vi "Fetch Waveform (Waveform Data Type)_mod.vi"(4 "Save data":bool, 6 "Channel name to save":string, 7 "tdms file":refnum<k34>, 8 "error in (no error)":errorcluster, 9 "Maximum Time (10000ms)":u32=10000, 10 "Channel (0: Channel 1)":u16(ring) items=["Channel 1", "Channel 2", "Channel 3", "Channel 4", "Math", "Reference 1", "Reference 2", "Reference 3", "Reference 4", "D0", "D1", "D2", "D3", "D4", "D5", "D6", "D7", "D8", "D9", "D10", "D11", "D12", "D13", "D14", "D15", "Amplitude", "Frequency", "Phase", "Normal", "Average", "Maximum Peak Hold", "Minimum Peak Hold"], 11 "VISA resource name":refnum<visa-resource-name>) -> (0 "error out":errorcluster, 2 "Waveform Data":waveform(dbl)(graph), 3 "VISA resource name out":refnum<visa-resource-name>, 5 "tdms file out":refnum<k34>)   [LabVIEW 2015]
doc: "Returns the waveform that an oscilloscope acquires for a channel you specify. An acquisition that you initiate before calling this VI generates the waveform.\n\nYou first enable channels with the Configure Channel VI. Then you use the Initiate VI to start an acquisition on the enabled channels. An oscilloscope concurrently acquires waveforms for these channels. You must call the Fetch Waveform VI separately to obtain waveforms for each enabled channel.\nHowever, you also can call the Read Waveform VI instead of using the above low-level VIs.\n\n<B>Note</B>: Use the Fetch Waveform VI only with other low-level VIs, such as the Initiate VI, the Abort VI, and the Fetch Waveform Measurement VI. High-level VIs, such as the Read Waveform VI, automatically incorporate the functions of the Initiate VI and the Fetch Waveform VI. The Fetch Waveform VI does not check the status of an instrument."
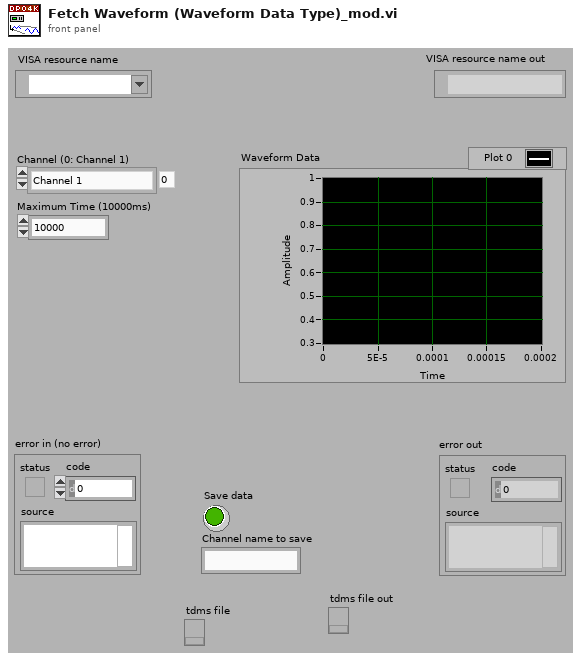
[diagram p1: front panel]
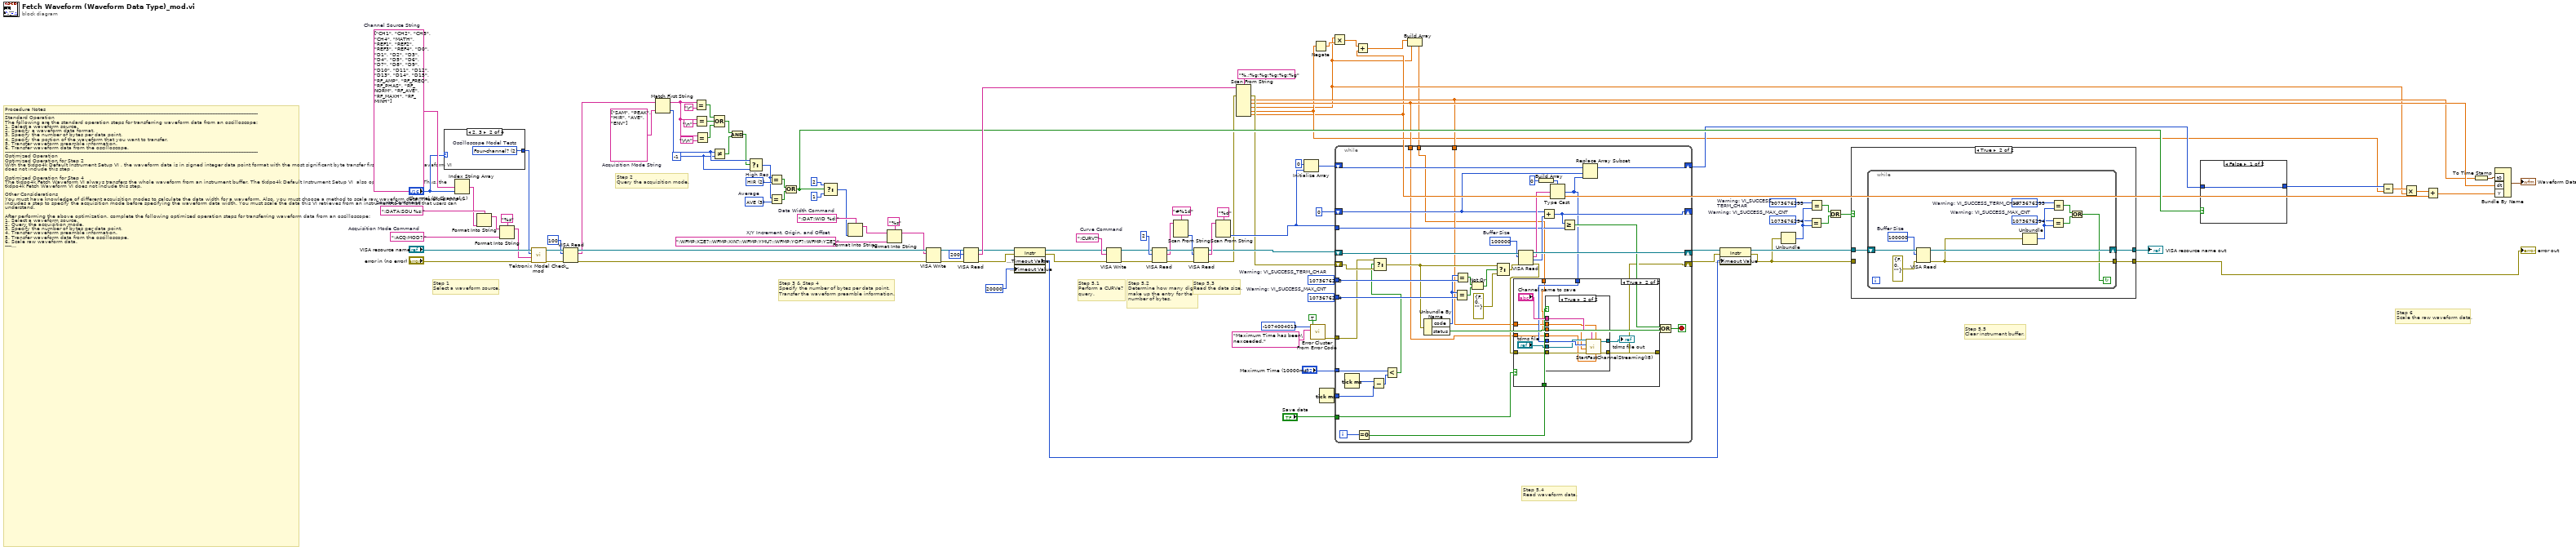
[diagram p0: block diagram]
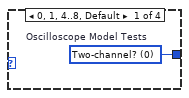
[diagram p2: hidden frame]
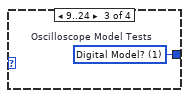
[diagram p3: hidden frame]
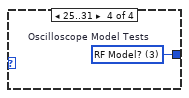
[diagram p4: hidden frame]
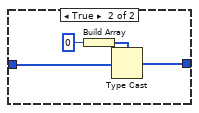
[diagram p5: hidden frame]
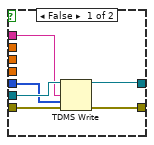
[diagram p8: hidden frame]
diagram:
  w51 = 1073676294  # Warning: VI_SUCCESS_MAX_CNT
  w52 = 1073676293  # Warning: VI_SUCCESS_TERM_CHAR
  w55 = 1073676294  # Warning: VI_SUCCESS_MAX_CNT
  w54 = 1073676293  # Warning: VI_SUCCESS_TERM_CHAR
  w64 = -1 ("y")
  w89 = ":CURV?"  # Curve Command
  w99 = ":DAT:WID %d;"  # Data Width Command
  w104 = u16 3 items=["SAM", "PEAK", "HIR", "AVE", "ENV"]  # Average
  w105 = u16 2 items=["SAM", "PEAK", "HIR", "AVE", "ENV"]  # High Res
  w76 = string[] ["SAM", "PEAK", "HIR", "AVE", "ENV"]  # Acquisition Mode String
  w98 = ":ACQ:MOD?;"  # Acquisition Mode Command
  w110 = string[] ["CH1", "CH2", "CH3", "CH4", "MATH", "REF1", "REF2", "REF3", "REF4", "D0", "D1", "D2", "D3", "D4", "D5", "D6", "D7", "D8", "D9", "D10", "D11", "D12", "D13", "D14", "D15", "RF_AMP", "RF_FREQ", "RF_PHAS", "RF_NORM", "RF_AVE", "RF_MAXH", "RF_MINH"]  # Channel Source String
  w109 = ":DATA:SOU %s;"  # Source Command
  w96 = ":WFMP:XZE?;:WFMP:XIN?;:WFMP:YMU?;:WFMP:YOF?;:WFMP:YZE?;"  # X/Y Increment, Origin, and Offset
  # "Step 6    \nScale the raw waveform data."
  # "Step 5.5    \nClear instrument buffer."
  # "Step 5.4   \nRead waveform data."
  # "Step 5.3      \nRead the data size."
  # "Step 5.2      \nDetermine how many digits\nmake up the entry for the \nnumber of bytes."
  # "Step 5.1      \nPerform a CURVe?\nquery."
  # "Step 3 & Step 4         \nSpecify the number of bytes per data point.\nTransfer the waveform preamble information."
  # "Step 2        \nQuery the acquisition mode."
  # "Step 1 \nSelect a waveform source."
  # "Procedure Notes\n-----------------------------------------------------------------------------------------------------------------------------------------------------------\nStandard Operation\nThe following are the standard operation steps for transferring waveform data from an oscilloscope:\n1. Select a waveform source.\n2. Specify a waveform data format.\n3. Specify the number of bytes per data point.\n4. Specify the portion of the waveform that you want to transfer.\n5. Transfer waveform preamble information.\n6. Transfer waveform data from the oscilloscope.\n-----------------------------------------------------------------------------------------------------------------------------------------------------------\nOptimized Operation\nOptimized Operation for Step 2\nWith the tkdpo4k Default Instrument Setup VI , the waveform data is in signed integer data point format with the most significant byte transfer first. Thus, the Fetch Waveform VI does not include this step . \n\nOptimized Operation for Step 4 \nThe tkdpo4k Fetch Waveform VI always transfers the whole waveform from an instrument buffer. The tkdpo4k Default Instrument Setup VI  also operates in this way. Thus, the tkdpo4k Fetch Waveform VI does not include this step. \n\nOther Considerations\nYou must have knowledge of different acquisition modes to calculate the data width for a waveform. Also, you must choose a method to scale raw waveform data. Therefore, this VI includes a step to specify the acquisition mode before specifying the waveform data width. You must scale the data this VI retrieves from an instrument to a format that users can understand.\n\nAfter performing the above optimization, complete the following optimized operation steps for transferring waveform data from an oscilloscope:\n1. Select a waveform source.\n2. Query the acquisition mode.\n3. Specify the number of bytes per data point.\n4. Transfer waveform preamble information.\n5. Transfer waveform data from the oscilloscope.\n6. Scale raw waveform data.\n-----------------------------------------------------------------------------------------------------------------------------------------------------------\nDetailed Steps\nThe following steps detail the behavior of this VI:\n1. Select a waveform source. \n2. Query and determine the acquisition mode. A correct determination is critical to steps 3 and 6.\n    -----------------------------------------------\n    Acquisition Mode |  Data Width   \n    -----------------------------------------------\n    Normal                       |   1                      \n    -----------------------------------------------\n    Peak Detect               |   1                      \n    -----------------------------------------------\n    Hi Res                        |   2                      \n    -----------------------------------------------\n    Envelope                   |   1                      \n    ----------------------------------------------- \n    Average                    |   2                      \n    -----------------------------------------------\n3. Specify the number of bytes per data point. For the Hi Res or Average acquisition modes, set the data width to 2. For all other acquisition modes, set the data width to 1.\n4. Transfer the waveform preamble information. Necessary preamble information includes XZero, XIncrement, YMultiplier, YOffset, and YZero. This VI uses XZero and XIncrement to configure the x-axis of output waveforms and uses YMultiplier, YOffset, and YZero to scale data values. This VI then parses the return string of the preamble query in step 6.\n5. Transfer waveform data from the oscilloscope.\n    5.1 Perform a CURVe? query.\n    5.2 Determine how many digits make up the entry for the number of bytes.\n    5.3 Read the data size.\n    5.4 Call the VISA Read VI repeatedly with a buffer size of 10000 until you obtain as much data as the data size specifies. Use      an 8-bit array to store the raw waveform data you obtain. \n    5.5 Continue reading the data remaining in the instrument buffer until the buffer is empty.\n6. Scale the raw waveform data.\n    6.1 Cast the waveform data to a 16-bit array if the data width is 2 . Split the waveform data into a minimum and a maximum data array if the acquisition mode is Peak Detect or Envelope. This VI skips this step if the data width is 1.\n    6.2 Parse the preamble information.\n    6.3 Scale the waveform data according to the following formula:\n          Data_Value_in_units = (Raw_Data_Value - YOffset) * YMultiplier + YZero\n          The resulting waveform data has a unit of volts.\n    6.4 Build a waveform graph."
  n1 = case shown="2, 3" "Channel (0: Channel 1)" {
    tunnel: [w111 w112 w113 w114] -> w14
    frame 0, 1, 4..8, Default {
      w111 = u16 0 items=["Two-channel?", "Digital Model?", "Four-channel?", "RF Model?"]  # Oscilloscope Model Tests
    }
    frame 2, 3 {
      w112 = u16 2 items=["Two-channel?", "Digital Model?", "Four-channel?", "RF Model?"]  # Oscilloscope Model Tests
    }
    frame 9..24 {
      w113 = u16 1 items=["Two-channel?", "Digital Model?", "Four-channel?", "RF Model?"]  # Oscilloscope Model Tests
    }
    frame 25..31 {
      w114 = u16 3 items=["Two-channel?", "Digital Model?", "Four-channel?", "RF Model?"]  # Oscilloscope Model Tests
    }
  }
  n2 = Index String Array(1:"Channel (0: Channel 1)", 2:w110) -> (0:w108:string)  [unwired: 1 in]
  n3 = Format Into String(format string=w109, w108) -> (resulting string=w107:string)  [unwired: 2 in, 1 out]
  n4 = Format Into String(format string="%s", initial string=w107, w98) -> (resulting string=w19:string)  [unwired: 1 in, 1 out]
  n5 = call "Tektronix Model Check_mod.vi"("error in (no error)"="error in (no error)", "Command String"=w19, "Oscilloscope Model Tests (3: RF Model?)"=w14, "VISA resource name"="VISA resource name") -> ("error out"=w17:errorcluster, "VISA resource name out"=w18:refnum<visa-resource-name>)  [unwired: 6 in]
  n6 = VISA Read(VISA resource name=w18, byte count=u32 100, error in (no error)=w17) -> (VISA resource name out=w95:refnum<visa-resource-name>, read buffer=w75:string, error out=w94:errorcluster)  [unwired: 1 out]
  n7 = Match First String(2:w76, 3:w75) -> (0:w65:i32, 1:w71:string)
  n8 = Equal?(x=w71, y="\r") -> (x = y?=w70:bool)
  n9 = Equal?(x=w71, y="\n") -> (x = y?=w69:bool)
  n10 = Equal?(x=w71, y="\r\n") -> (x = y?=w68:bool)
  n11 = Not Equal?(x=w65, y=w64) -> (x != y?=w66:bool)
  n12 = Compound Arithmetic op=OR(w70, w69, w68) -> (w67:bool)
  n13 = And(x=w67, y=w66) -> (x .and. y?=w63:bool)
  n14 = Select(t=w65, s=w63, f=w64) -> (s? t:f=w50:i32)
  n15 = Equal?(x=w50, y=w105) -> (x = y?=w103:bool)
  n16 = Equal?(x=w50, y=w104) -> (x = y?=w102:bool)
  n17 = Or(x=w103, y=w102) -> (x .or. y?=w49:bool)
  n18 = Select(t=2 ("f"), s=w49, f=1) -> (s? t:f=w79:i32)
  n19 = Format Into String(format string=w99, w79) -> (resulting string=w93:string)  [unwired: 2 in, 1 out]
  n20 = Format Into String(format string="%s", initial string=w93, w96) -> (resulting string=w80:string)  [unwired: 1 in, 1 out]
  n21 = VISA Write(VISA resource name=w95, write buffer=w80, error in (no error)=w94) -> (VISA resource name out=w91:refnum<visa-resource-name>, error out=w90:errorcluster)  [unwired: 1 out]
  n22 = VISA Read(VISA resource name=w91, byte count=u32 200, error in (no error)=w90) -> (VISA resource name out=w28:refnum<visa-resource-name>, read buffer=w78:string, error out=w27:errorcluster)  [unwired: 1 out]
  n23 = property class="Instr"(reference=w28, error in=w27, "General Settings:Timeout Value"=u32 20000) -> (reference out=w26:refnum<visa-resource-name>, error out=w24:errorcluster, "General Settings:Timeout Value"=w37:u32)
  n24 = VISA Write(VISA resource name=w26, write buffer=w89, error in (no error)=w24) -> (VISA resource name out=w25:refnum<visa-resource-name>, error out=w23:errorcluster)  [unwired: 1 out]
  n25 = VISA Read(VISA resource name=w25, byte count=u32 2, error in (no error)=w23) -> (VISA resource name out=w86:refnum<visa-resource-name>, read buffer=w84:string, error out=w85:errorcluster)  [unwired: 1 out]
  n26 = Scan From String(format string="#%1d", input string=w84) -> (output 1=w83:i32)  [unwired: 3 in, 3 out]
  n27 = VISA Read(VISA resource name=w86, byte count=w83, error in (no error)=w85) -> (VISA resource name out=w22:refnum<visa-resource-name>, read buffer=w81:string, error out=w11:errorcluster)  [unwired: 1 out]
  n28 = Scan From String(format string="%d", input string=w81) -> (output 1=w62:i32)  [unwired: 3 in, 3 out]
  n29 = Scan From String(format string="%.;%g;%g;%g;%g;%g", input string=w78, error in=w11) -> (error out=w10:errorcluster, output 1=w8:dbl, output 2=w9:dbl, output 3=w2:dbl, output 4=w6:dbl, output 5=w4:dbl)  [unwired: 6 in, 2 out]
  n30 = Initialize Array(i8 0 ("element"), w62) -> (w60:i8[])
  n31 = call <vilib>:"Error Cluster From Error Code.vi"("show call chain? (False)"=TRUE, "error message (\"\")"="Maximum Time has been\nexceeded." ("error message (\"\")"), "error code (0)"=-1074004013) -> ("error out"=w29:errorcluster)  [unwired: 6 in]
  n32 = Negate(x=w6) -> (-x=w7:dbl)
  n33 = Tick Count (ms)() -> (millisecond timer value=w34:u32)
  n34 = Multiply(x=w2, y=w7) -> (x*y=w5:dbl)
  n35 = Add(x=w5, y=w4) -> (x+y=w3:dbl)
  n36 = Build Array(w3, w2) -> (w1:dbl[])
  n37 = while {
    shift-right: [w152] -> w39
    shift-left: w22 -> [w154]
    shift-right: [w119] -> w38
    shift-left: w10 -> [w126]
    shift-right: [w148] -> w48
    shift-left: w60 -> [w149]
    tunnel: w62 -> [w145]
    shift-right: [w143] -> _
    shift-left: 0 -> [w144]
    tunnel: w52 -> [w137]
    tunnel: w51 -> [w136]
    tunnel: w34 -> [w130]
    tunnel: "Maximum Time (10000ms)" -> [w128]
    tunnel: w29 -> [w125]
    tunnel: "Save data" -> [w121]
    tunnel: w9 -> [w117]
    tunnel: w8 -> [w116]
    tunnel: w1 -> [w115]
    i -> [w123]
    stop <- w142 stop-if-true
    w153 = 100000  # Buffer Size
    n38 = Tick Count (ms)() -> (millisecond timer value=w131:u32)
    n39 = Equal To 0?(x=w123) -> (x = 0?=w122:bool)
    n40 = Subtract(x=w131, y=w130) -> (x-y=w129:u32)
    n41 = Less?(x=w128, y=w129) -> (x < y?=w124:bool)
    n42 = Select(t=w125, s=w124, f=w126) -> (s? t:f=w127:errorcluster)
    n43 = Unbundle By Name(w127) -> ("code"=w135:i32, "status"=w139:bool)
    n44 = Equal?(x=w135, y=w136) -> (x = y?=w133:bool)
    n45 = Equal?(x=w135, y=w137) -> (x = y?=w134:bool)
    n46 = Not Or(1:w133, 2:w134) -> (0:w132:bool)
    n47 = Select(t=w127, s=w132, f=errorcluster {"status"=FALSE, "code"=0, "source"=""} ("error in (no error)")) -> (s? t:f=w138:errorcluster)
    n48 = VISA Read(VISA resource name=w154, byte count=w153, error in (no error)=w138) -> (VISA resource name out=w152:refnum<visa-resource-name>, read buffer=w147:string, return count=w146:u32, error out=w120:errorcluster)
    n49 = Build Array(i8 0) -> (w151:i8[])
    n50 = Add(x=w144, y=w146) -> (x+y=w143:u32)
    n51 = Type Cast(type=w151, x=w147) -> (*(type *) &x=w118:i8[])
    n52 = case shown="True" w121 {
      tunnel: w122 -> [_ w164]
      tunnel: w120 -> [w155 w163]
      tunnel: [w155 w162] -> w119
      tunnel: w118 -> [_ w160]
      tunnel: w117 -> [_ w159]
      tunnel: w116 -> [_ w158]
      tunnel: w115 -> [_ w157]
      frame False {
      }
      frame True {
        n53 = case shown="True" w164 {
          tunnel: w163 -> [w171 w180]
          tunnel: [w170 w179] -> w162
          tunnel: w160 -> [w166 w178]
          tunnel: "tdms file" -> [w169 w177]
          tunnel: "Channel name to save" -> [w167 w176]
          tunnel: w158 -> [_ w175]
          tunnel: w159 -> [_ w174]
          tunnel: w157 -> [_ w173]
          tunnel: [w168 w172] -> w156
          frame False {
            n54 = TDMS Write(0:w169, 7:w167, 9:w166, 11:w171) -> (4:w168:refnum<k34>, 15:w170:errorcluster)  [unwired: 2 in, 2 out]
          }
          frame True {
            n55 = call "StartFastChannelStreaming(I8).vi"("dt"=w174, "t0"=w175, "channel name(s) in (Untitled)"=w176, "error in (no error)"=w180, "Scaling coefficients"=w173, "Data"=w178, "tdms file"=w177) -> ("error out"=w179:errorcluster, "tdms file out"=w172:refnum<k34>)  [unwired: 3 in]
          }
        }
        "tdms file out" <- w156
      }
    }
    n56 = Greater Or Equal?(x=w143, y=w145) -> (x >= y?=w141:bool)
    n57 = Replace Array Subset(array=w149, new element=w118, index=w144) -> (w148:i8[])
    n58 = Compound Arithmetic op=OR(w141, w139) -> (w142:bool)
  }
  n59 = property class="Instr"(reference=w39, error in=w38, "General Settings:Timeout Value"=w37) -> (reference out=w36:refnum<visa-resource-name>, error out=w35:errorcluster)
  n60 = Unbundle(w35) -> ("code"=w56:i32)  [unwired: 2 out]
  n61 = Equal?(x=w55, y=w56) -> (x = y?=w58:bool)
  n62 = Equal?(x=w54, y=w56) -> (x = y?=w59:bool)
  n63 = Or(x=w59, y=w58) -> (x .or. y?=w57:bool)
  n64 = case shown="True" w57 {
    tunnel: w36 -> [w182 w185]
    tunnel: w35 -> [w181 _]
    tunnel: [w182 w184] -> w77
    tunnel: [w181 w183] -> w12
    frame False {
    }
    frame True {
      n65 = while {
        shift-right: [w195] -> w184
        shift-left: w185 -> [w196]
        tunnel: [w188] -> w183
        stop <- w187 continue-if-true
        w190 = 1073676294  # Warning: VI_SUCCESS_MAX_CNT
        w189 = 1073676293  # Warning: VI_SUCCESS_TERM_CHAR
        w194 = u32 100000  # Buffer Size
        n66 = VISA Read(VISA resource name=w196, byte count=w194, error in (no error)=errorcluster {"status"=FALSE, "code"=0, "source"=""}) -> (VISA resource name out=w195:refnum<visa-resource-name>, error out=w188:errorcluster)  [unwired: 2 out]
        n67 = Unbundle(w188) -> ("code"=w191:i32)  [unwired: 2 out]
        n68 = Equal?(x=w190, y=w191) -> (x = y?=w192:bool)
        n69 = Equal?(x=w189, y=w191) -> (x = y?=w193:bool)
        n70 = Or(x=w193, y=w192) -> (x .or. y?=w187:bool)
      }
    }
  }
  "error out" <- w12
  "VISA resource name out" <- w77
  n71 = case shown="False" w49 {
    tunnel: w48 -> [w197 w199]
    tunnel: [w197 w198] -> w42
    frame False {
    }
    frame True {
      n72 = Build Array(i16 0 ("element")) -> (w200:i16[])
      n73 = Type Cast(type=w200, x=w199) -> (*(type *) &x=w198:i16[])
    }
  }
  n74 = Subtract(x=w42, y=w6) -> (x-y=w46:dbl[])
  n75 = Multiply(x=w46, y=w2) -> (x*y=w45:dbl[])
  n76 = Add(x=w45, y=w4) -> (x+y=w44:dbl[])
  n77 = To Time Stamp(1:w8) -> (0:w43:timestamp)
  n78 = Bundle By Name("t0"=w43, "dt"=w9, "Y"=w44) -> (→"Waveform Data":waveform(dbl))  [unwired: 1 in]
